vi "solar_msg Q EnQ (Name).vi"(5 "Handshake? (F)":bool, 6 "HS Timeout ms (60000)":u32=60000, 7 "Priority (Normal)":enum8{"Normal", "Priority", "IgnoreIfExists"}(ring), 8 "error in (no error)":errorcluster, 9 "CMD_DATA":variant, 10 "CMD":string, 11 "Target":string) -> (0 "error out":errorcluster, 1 "TLM_DATA":variant, 2 "TLM":string, 3 "TLM Timed Out?":bool)   [LabVIEW 2018]
doc: "This enqueues a message to the <b>Target</b>. If <b>Handshake</b> is true this creates a handshake reference ('HS' queue) and waits for the handshake response. Set <b>Priority</b> to enqueue to the back (Normal), front (Priority) or filtered (Ignore If Exists)."
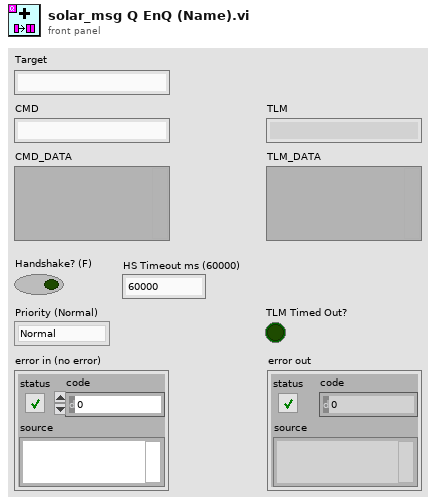
[diagram p1: front panel]
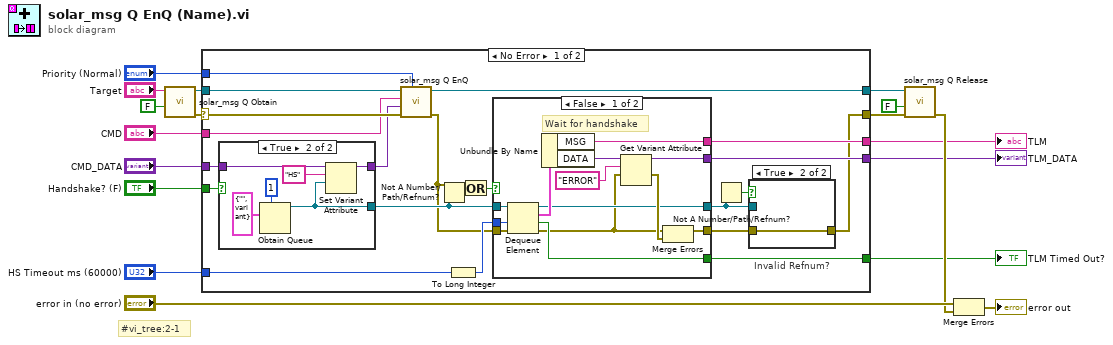
[diagram p0: block diagram]
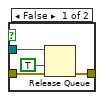
[diagram p2: hidden frame]
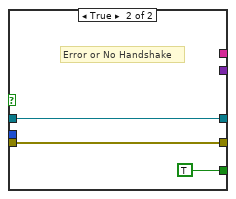
[diagram p3: hidden frame]
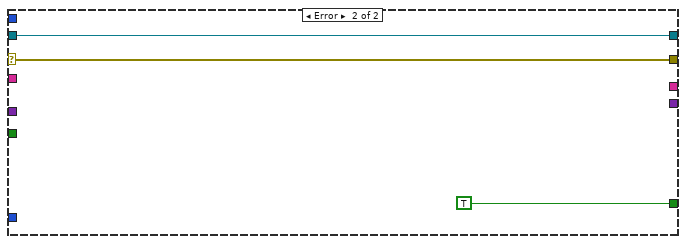
[diagram p5: hidden frame]
diagram:
  # "#vi_tree:2-1"
  n1 = call "solar_msg Q Obtain.vi"("Create If Not Found? (T)"=FALSE, "Queue Name (unnamed)"="Target") -> ("error out"=w18:errorcluster, "Queue"=w17:refnum<queue>)  [unwired: 7 in, 1 out]
  n2 = case shown="No Error" w18 {
    selector: w18 -> [w39 w70]
    tunnel: w17 -> [w38 w69]
    tunnel: [w19 w70] -> w16
    tunnel: [w37 w69] -> w15
    tunnel: "Priority (Normal)" -> [w36 _]
    tunnel: "CMD" -> [w35 _]
    tunnel: "Handshake? (F)" -> [w34 _]
    tunnel: "CMD_DATA" -> [w32 _]
    tunnel: "HS Timeout ms (60000)" -> [w28 _]
    tunnel: [w27 TRUE ("timed out?")] -> w3
    tunnel: [w25 _] -> w2
    tunnel: [w24 _] -> w1
    frame No Error {
      n3 = case shown="True" w34 {
        tunnel: [w61 w66] -> w33
        tunnel: w32 -> [w61 w67]
        tunnel: [_ w62] -> w29
        frame False {
          # "No Handshake"
        }
        frame True {
          n4 = Obtain Queue(max queue size (-1, unlimited)=1, element data type=cluster{"MSG":string, "DATA":variant} {"MSG"="", "DATA"=variant} ("MSG")) -> (queue out=w62:refnum<queue>)  [unwired: 3 in, 2 out]
          n5 = Set Variant Attribute(Variant=w67, name="HS", value=w62) -> (Variant out=w66:variant)  [unwired: 1 in, 2 out]
        }
      }
      n6 = call "solar_msg Q EnQ.vi"("Priority (Normal)"=w36, "error in (no error)"=w39, "CMD_DATA (Last)"=w33, "CMD (Last)"=w35, "Queue in"=w38) -> ("error out"=w26:errorcluster, "Queue out"=w37:refnum<queue>)  [unwired: 4 in, 1 out]
      n7 = Not A Number/Path/Refnum?(number/path/refnum=w29) -> (NaN/Path/Refnum?=w23:bool)
      n8 = To Long Integer(number=w28) -> (32bit integer=w31:i32)
      n9 = Or(x=w26, y=w23) -> (x .or. y?=w30:bool)
      n10 = case shown="False" w30 {
        tunnel: w29 -> [w57 w58]
        tunnel: w26 -> [w56 w59]
        tunnel: w31 -> [w55 _]
        tunnel: [w49 w59] -> w22
        tunnel: [w54 TRUE ("timed out?")] -> w27
        tunnel: [w48 _] -> w25
        tunnel: [w47 _] -> w24
        tunnel: [w46 w58] -> w20
        frame False {
          # "Wait for handshake"
          n11 = Dequeue Element(queue=w57, timeout in ms (-1)=w55, error in (no error)=w56) -> (queue out=w46:refnum<queue>, element=w50:cluster{"MSG":string, "DATA":variant}, timed out?=w54:bool, error out=w45:errorcluster)
          n12 = Unbundle By Name(w50) -> ("MSG"=w48:string, "DATA"=w53:variant)
          n13 = Get Variant Attribute(Variant=w53, name="ERROR", default value (empty Variant)=w45) -> (duplicate Variant=w47:variant, value=w52:errorcluster)  [unwired: 1 in, 2 out]
          n14 = Merge Errors(w45, w52) -> (w49:errorcluster)
        }
        frame True {
          # "Error or No Handshake"
        }
      }
      n15 = Not A Number/Path/Refnum?(number/path/refnum=w20) -> (NaN/Path/Refnum?=w21:bool)
      n16 = case "Invalid Refnum?" shown="True" w21 {
        tunnel: w20 -> [w41 _]
        tunnel: w22 -> [w43 w44]
        tunnel: [w42 w44] -> w19
        frame False {
          n17 = Release Queue(queue=w41, force destroy? (F)=TRUE, error in (no error)=w43) -> (error out=w42:errorcluster)  [unwired: 2 out]
        }
        frame True {
        }
      }
    }
    frame Error {
    }
  }
  "TLM Timed Out?" <- w3
  "TLM" <- w2
  "TLM_DATA" <- w1
  n18 = call "solar_msg Q Release.vi"("error in (no error)"=w16, "Force Destroy? (F)"=FALSE, "Queue"=w15) -> ("error out"=w6:errorcluster)  [unwired: 6 in, 2 out]
  n19 = Merge Errors("error in (no error)", w6) -> (→"error out":errorcluster)
